vi "LV2G_FilterPort.vi"(7 "Operation":T2, 8 "error in (no error)":errorcluster, 11 "Modbus485":T1={"Port"="", "baud rate"=9600, "data bits"=8, "stop bits"=10, "parity"=enum."None", "flow control"=0, "Timeout"=9600} {"flow control" items=["None", "XON/XOFF", "RTS/CTS", "XON/XOFF & RTS/CTS", "DTR/DSR", "XON/XOFF & DTR/DSR"]; "stop bits" items=["1.0"=10, "1.5"=15, "2.0"=20]; "data bits" min=5 max=8 step=1}) -> (0 "error out":errorcluster, 3 "Modbus485 Out":T1={"Port"="", "baud rate"=9600, "data bits"=8, "stop bits"=10, "parity"=enum."None", "flow control"=0, "Timeout"=9600} {"flow control" items=["None", "XON/XOFF", "RTS/CTS", "XON/XOFF & RTS/CTS", "DTR/DSR", "XON/XOFF & DTR/DSR"]; "stop bits" items=["1.0"=10, "1.5"=15, "2.0"=20]; "data bits" min=5 max=8 step=1})   [LabVIEW 2018]
uses:
  <vilib>/Utility/config.llb/NI_LVConfig.lvlib
  <vilib>/Utility/config.llb/Read Key (String).vi
  <vilib>/Utility/config.llb/Write Key (String).vi
  Strict Type Controls/Settings Operation.ctl
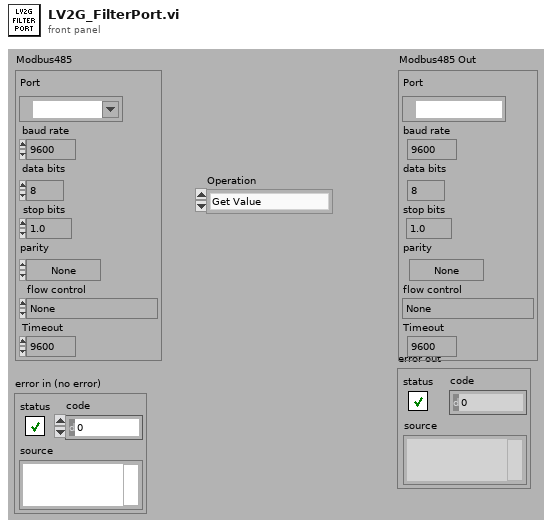
[diagram p1: front panel]
types:
  T1 = cluster{"Port":refnum<visa-resource-name>, "baud rate":u32, "data bits":u16, "stop bits":u16, "parity":enum16{"None", "Odd", "Even", "Mark", "Space"}, "flow control":u16, "Timeout":u32}
  T2 = typedef "Settings Operation.ctl" = enum8{"Get Value", "Set Value", "Read File", "Write File", "Write Stored Value"}
  T3 = typedef "NI_LVConfig.lvlib/Config Data RefNum.ctl" = refnum<k1>
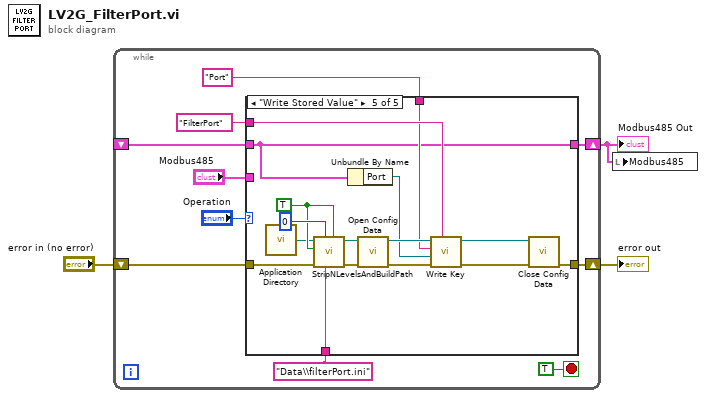
[diagram p0: block diagram]
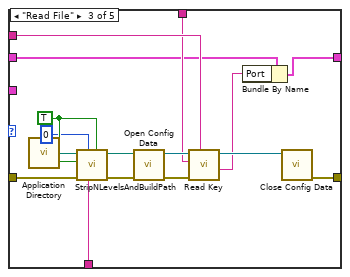
[diagram p4: hidden frame]
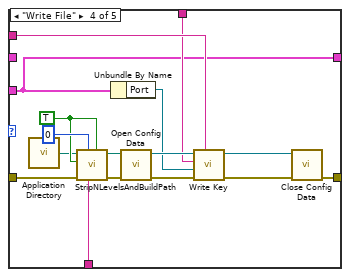
[diagram p5: hidden frame]
diagram:
  n1 = while {
    shift-right: [w12] -> w1
    shift-left: _ -> [w13]
    shift-right: [w10] -> w2
    shift-left: "error in (no error)" -> [w11]
    stop <- TRUE stop-if-true
    n2 = case shown="\"Write Stored Value\"" "Operation" {
      tunnel: w13 -> [w15 _ w20 _ w50]
      tunnel: [w15 w17 w19 w37 w50] -> w12
      tunnel: "Modbus485" -> [_ w17 _ w37 _]
      tunnel: w11 -> [w14 w16 w32 w48 w64]
      tunnel: [w14 w16 w33 w49 w65] -> w10
      tunnel: "Data\\filterPort.ini" ("Build Path") -> [_ _ w29 w47 w63]
      tunnel: "FilterPort" ("section") -> [_ _ w24 w39 w55]
      tunnel: "Port" ("section") -> [_ _ w22 w38 w54]
      frame "Get Value", Default {
      }
      frame "Set Value" {
      }
      frame "Read File" {
        w27 = TRUE ("Is File?")
        n3 = call <vilib>:"Application Directory.vi"() -> ("Application Directory"=w28:path)
        n4 = call "StripNLevelsAndBuildPath.vi"("Create Folders"=w27, "Build Path"=w29, "Strip Levels"=0, "error in(no error)"=w32, "Is File"=w27, "Path In"=w28) -> ("error out"=w31:errorcluster, "Path Out"=w30:path)  [unwired: 4 in]
        n5 = call <vilib>:"Open Config Data.vi"("error in (no error)"=w31, "configuration file path"=w30) -> ("error out"=w23:errorcluster, "refnum"=w25:T3)  [unwired: 7 in, 1 out]
        n6 = call-poly <vilib>:"Read Key.vi"("section"=w24, "error in (no error)"=w23, "key"=w22, "refnum"=w25) -> ("value"=w18:string, "refnum out"=w21:T3)  [unwired: 4 in, 2 out]
        n7 = Bundle By Name(cluster=w20, "Port"=w18) -> (w19:T1)
        n8 = call <vilib>:"Close Config Data.vi"("refnum"=w21) -> ("error out"=w33:errorcluster)  [unwired: 2 in, 8 out]
      }
      frame "Write File" {
        w45 = TRUE ("Is File?")
        n9 = call <vilib>:"Application Directory.vi"() -> ("Application Directory"=w44:path)
        n10 = call "StripNLevelsAndBuildPath.vi"("Create Folders"=w45, "Build Path"=w47, "Strip Levels"=0, "error in(no error)"=w48, "Is File"=w45, "Path In"=w44) -> ("error out"=w43:errorcluster, "Path Out"=w42:path)  [unwired: 4 out]
        n11 = Unbundle By Name(w37) -> ("Port"=w36:refnum<visa-resource-name>)
        n12 = call <vilib>:"Open Config Data.vi"("error in (no error)"=w43, "configuration file path"=w42) -> ("error out"=w35:errorcluster, "refnum"=w41:T3)  [unwired: 7 in, 1 out]
        n13 = call-poly <vilib>:"Write Key.vi"("section"=w39, "error in (no error)"=w35, "value"=w36, "key"=w38, "refnum"=w41) -> ("error out"=w34:errorcluster, "refnum out"=w40:T3)  [unwired: 4 in, 1 out]
        n14 = call <vilib>:"Close Config Data.vi"("error in (no error)"=w34, "refnum"=w40) -> ("error out"=w49:errorcluster)  [unwired: 1 in, 8 out]
      }
      frame "Write Stored Value" {
        w61 = TRUE ("Is File?")
        n15 = call <vilib>:"Application Directory.vi"() -> ("Application Directory"=w60:path)
        n16 = call "StripNLevelsAndBuildPath.vi"("Create Folders"=w61, "Build Path"=w63, "Strip Levels"=0, "error in(no error)"=w64, "Is File"=w61, "Path In"=w60) -> ("error out"=w59:errorcluster, "Path Out"=w58:path)  [unwired: 4 out]
        n17 = Unbundle By Name(w50) -> ("Port"=w53:refnum<visa-resource-name>)
        n18 = call <vilib>:"Open Config Data.vi"("error in (no error)"=w59, "configuration file path"=w58) -> ("error out"=w52:errorcluster, "refnum"=w57:T3)  [unwired: 7 in, 1 out]
        n19 = call-poly <vilib>:"Write Key.vi"("section"=w55, "error in (no error)"=w52, "value"=w53, "key"=w54, "refnum"=w57) -> ("error out"=w51:errorcluster, "refnum out"=w56:T3)  [unwired: 4 in, 1 out]
        n20 = call <vilib>:"Close Config Data.vi"("error in (no error)"=w51, "refnum"=w56) -> ("error out"=w65:errorcluster)  [unwired: 1 in, 8 out]
      }
    }
  }
  "error out" <- w2
  "Modbus485 Out" <- w1
  n21 = local write "Modbus485"(w1) -> ()
